vi "bofabthetaphi.vi"(8 "phi":dbl[](array[numeric]), 9 "theta":dbl, 10 "b":dbl, 11 "a":dbl) -> (0 "dB dtheta":T1, 1 "dB db":T2, 2 "dB da":T3, 3 "B":cluster{"Bx":dbl[], "By":dbl[], "Bz":dbl[]})   [LabVIEW 2017]
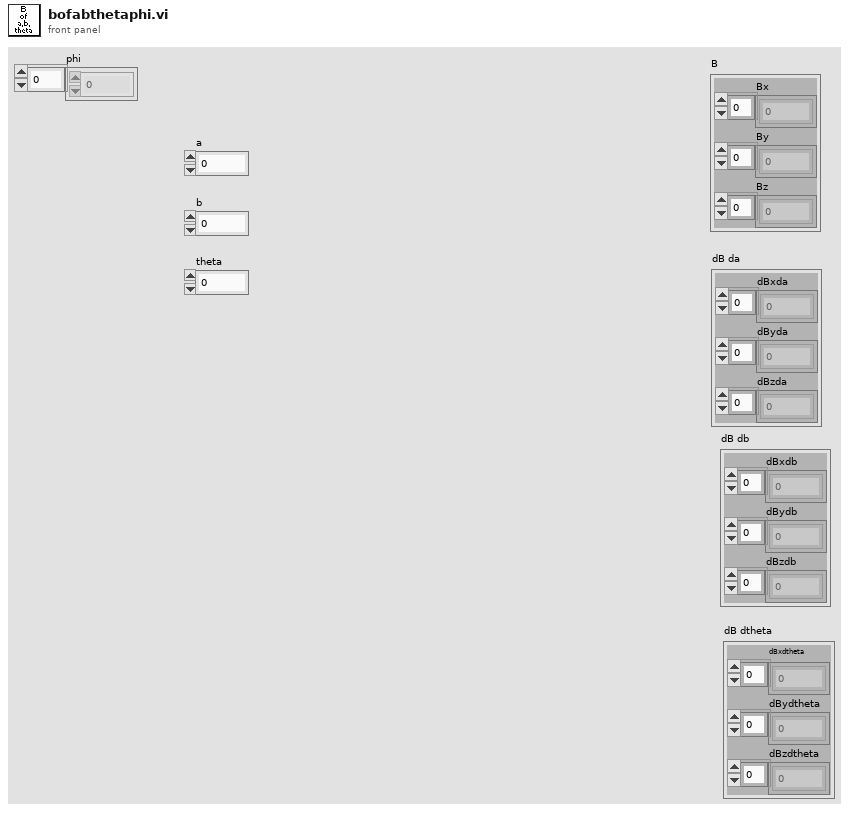
[diagram p1: front panel]
types:
  T1 = cluster{"dBxdtheta":dbl[], "dBydtheta":dbl[], "dBzdtheta":dbl[]}
  T2 = cluster{"dBxdb":dbl[], "dBydb":dbl[], "dBzdb":dbl[]}
  T3 = cluster{"dBxda":dbl[], "dByda":dbl[], "dBzda":dbl[]}
  T4 = cluster{"dBxdy":dbl[], "dBydy":dbl[], "dBzdy":dbl[]}
  T5 = cluster{"dBxdx":dbl[], "dBydx":dbl[], "dBzdx":dbl[]}
  T6 = cluster{"dfda":dbl[], "dfda":dbl[], "dfda":dbl[]}
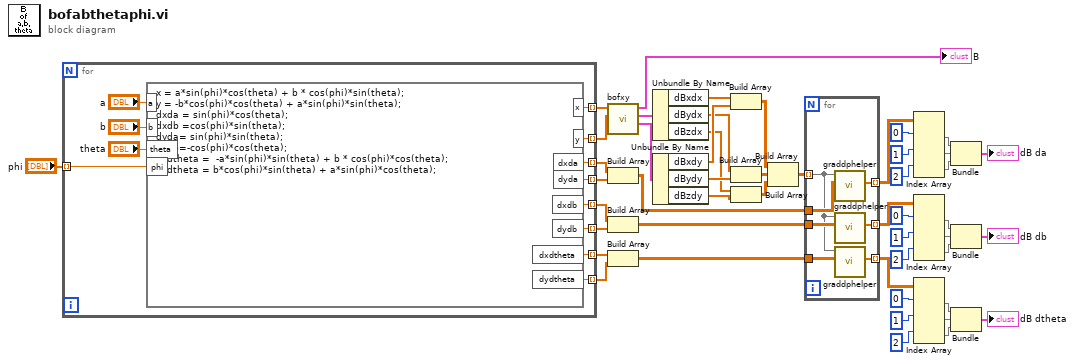
[diagram p0: block diagram]
diagram:
  n1 = for {
    tunnel: "phi" -> [w61] mode=indexing
    tunnel: [w57] -> w48 mode=indexing
    tunnel: [w56] -> w47 mode=indexing
    tunnel: [w55] -> w44 mode=indexing
    tunnel: [w54] -> w43 mode=indexing
    tunnel: [w53] -> w42 mode=indexing
    tunnel: [w52] -> w41 mode=indexing
    tunnel: [w51] -> w40 mode=indexing
    tunnel: [w50] -> w39 mode=indexing
    n2 = formula code="x = a*sin(phi)*cos(theta) + b * cos(phi)*sin(theta);\ny = -b*cos(phi)*cos(theta) + a*sin(phi)*sin(theta);\ndxda = sin(phi)*cos(theta);\ndxdb =cos(phi)*sin(theta);\ndyda= sin(phi)*sin(theta);\ndydb=-cos(phi)*cos(theta);\ndxdtheta =  -a*sin(phi)*sin(theta) + b * cos(phi)*cos(theta);\ndydtheta = b*cos(phi)*sin(theta) + a*sin(phi)*cos(theta);"("a"="a", "b"="b", "theta"="theta", "phi"=w61) -> ("x"=w57:dbl, "y"=w56:dbl, "dxda"=w55:dbl, "dyda"=w54:dbl, "dxdb"=w53:dbl, "dydb"=w52:dbl, "dxdtheta"=w51:dbl, "dydtheta"=w50:dbl)
  }
  n3 = call "bofxy.vi"("Y"=w47, "X"=w48) -> ("dB dy"=w45:T4, "dB dx"=w46:T5, "B"=→"B":cluster{"Bx":dbl[], "By":dbl[], "Bz":dbl[]})  [unwired: 7 in]
  n4 = Build Array(w44, w43) -> (w28:dbl[][])
  n5 = Build Array(w42, w41) -> (w27:dbl[][])
  n6 = Build Array(w40, w39) -> (w26:dbl[][])
  n7 = Unbundle By Name(w46) -> ("dBxdx"=w38:dbl[], "dBydx"=w36:dbl[], "dBzdx"=w34:dbl[])
  n8 = Unbundle By Name(w45) -> ("dBxdy"=w37:dbl[], "dBydy"=w35:dbl[], "dBzdy"=w33:dbl[])
  n9 = Build Array(w38, w37) -> (w32:dbl[][])
  n10 = Build Array(w36, w35) -> (w31:dbl[][])
  n11 = Build Array(w34, w33) -> (w30:dbl[][])
  n12 = Build Array(w32, w31, w30) -> (w29:dbl[][][])
  n13 = for {
    tunnel: w29 -> [w65] mode=indexing
    tunnel: w28 -> [w68]
    tunnel: w27 -> [w67]
    tunnel: w26 -> [w66]
    tunnel: [w64] -> w25 mode=indexing
    tunnel: [w63] -> w10 mode=indexing
    tunnel: [w62] -> w2 mode=indexing
    n14 = call "graddphelper.vi"("dxda,dyda"=w68, "dfdx,dfdy"=w65) -> ("dfda"=w64:dbl[])  [unwired: 9 in]
    n15 = call "graddphelper.vi"("dxda,dyda"=w67, "dfdx,dfdy"=w65) -> ("dfda"=w63:dbl[])  [unwired: 9 in]
    n16 = call "graddphelper.vi"("dxda,dyda"=w66, "dfdx,dfdy"=w65) -> ("dfda"=w62:dbl[])  [unwired: 9 in]
  }
  n17 = Index Array(array=w25, index (row) #1=0, index (row) #2=1, index (row) #3=2 ("index (row)")) -> (element #1=w21:dbl[], element #2=w20:dbl[], element #3=w19:dbl[])  [unwired: 3 in]
  n18 = Index Array(array=w10, index (row) #1=0, index (row) #2=1, index (row) #3=2 ("index (row)")) -> (element #1=w14:dbl[], element #2=w13:dbl[], element #3=w12:dbl[])  [unwired: 3 in]
  n19 = Index Array(array=w2, index (row) #1=0, index (row) #2=1, index (row) #3=2 ("index (row)")) -> (element #1=w6:dbl[], element #2=w5:dbl[], element #3=w4:dbl[])  [unwired: 3 in]
  n20 = Bundle("dfda"=w21, "dfda"=w20, "dfda"=w19) -> (→"dB da":T6)  [unwired: 1 in]
  n21 = Bundle("dfda"=w14, "dfda"=w13, "dfda"=w12) -> (→"dB db":T6)  [unwired: 1 in]
  n22 = Bundle("dfda"=w6, "dfda"=w5, "dfda"=w4) -> (→"dB dtheta":T6)  [unwired: 1 in]
